vi "SysDef.Search.vi"   [LabVIEW 2027, in "Advanced System Definition.lvlib"]
uses:
  Advanced System Definition.lvlib
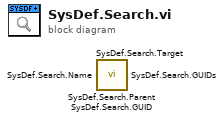
[diagram p0: block diagram]
diagram:
  n1 = call <vilib>:"SysDef.Search.Parent.vi"() -> ()  [unwired: 8 in, 4 out]
  n2 = call <vilib>:"SysDef.Search.Target.vi"() -> ()  [unwired: 8 in, 4 out]
  n3 = call <vilib>:"SysDef.Search.Name.vi"() -> ()  [unwired: 8 in, 4 out]
  n4 = call <vilib>:"SysDef.Search.GUIDs.vi"() -> ()  [unwired: 8 in, 4 out]
  n5 = call <vilib>:"SysDef.Search.GUID.vi"() -> ()  [unwired: 8 in, 4 out]
